vi "Read Subscriber.vi"(8 "error in (no error)":errorcluster, 11 "Device Connector MSG in":refnum<class "Device Connector MSG.lvclass">) -> (0 "error out":errorcluster, 2 "Subscriber.lvclass":refnum<class "Subscriber.lvclass">, 3 "Device Connector MSG out":refnum<class "Device Connector MSG.lvclass">)   [LabVIEW 2019, in "Device Connector MSG.lvclass"]
uses:
  Device Connector MSG.lvclass
  Ancestor Class/Subscriber/Subscriber.lvclass
  Device Connector MSG.lvclass/Device Connector MSG.ctl
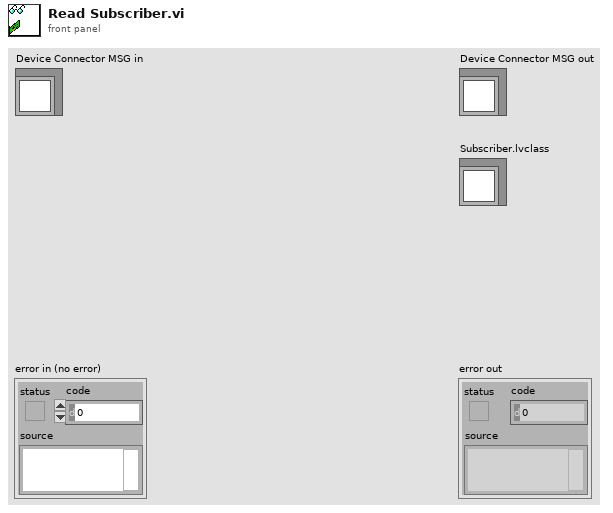
[diagram p1: front panel]
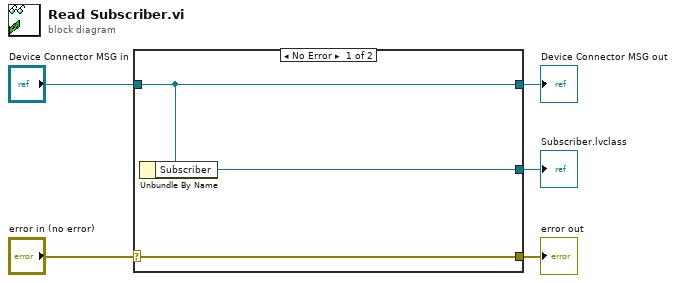
[diagram p0: block diagram]
diagram:
  n1 = case shown="No Error" "error in (no error)" {
    selector: "error in (no error)" -> [w8 w9]
    tunnel: [w8 w9] -> w4
    tunnel: [w7 w10] -> w2
    tunnel: "Device Connector MSG in" -> [w7 w10]
    tunnel: [w6 _] -> w1
    frame No Error {
      n2 = Unbundle By Name(w7) -> ("Subscriber"=w6:refnum<class "Subscriber.lvclass">)
    }
    frame Error {
    }
  }
  "error out" <- w4
  "Device Connector MSG out" <- w2
  "Subscriber.lvclass" <- w1
